vi "WSVCAP SHL Host LL SPI Set Configuration Parameters.vi"(0 "I2C_Clock Divider":u32=20, 11 "error in (no error)":errorcluster) -> (15 "error out":errorcluster)   [LabVIEW 2012]
uses:
  Type Defs/WSVCAP SHL Top Level Control Enum.ctl
  Type Defs/WSVCAP SHL Top Level Control Operation Enum.ctl
  Type Defs/WSVCAP SHL State.ctl
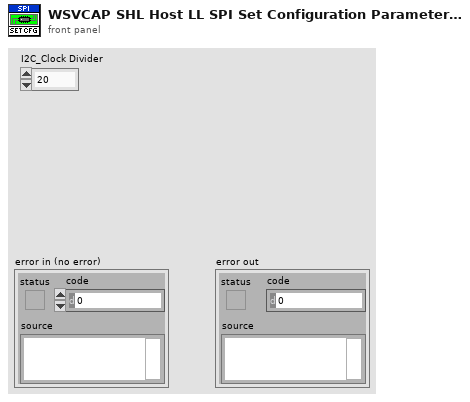
[diagram p1: front panel]
types:
  T1 = typedef "WSVCAP SHL State.ctl" = enum8{"Idle", "Transfer Data"}
  T2 = typedef "WSVCAP SHL Top Level Control Operation Enum.ctl" = enum16{"Initialize", "Set Control", "Read Control", "Close"}
  T3 = typedef "WSVCAP SHL Top Level Control Enum.ctl" = enum16{"Start", "Cmd", "Transaction", "Wait Ticks", "Socket Mask", "UUT Set", "Slave Address", "Sub Address", "Bytes to Write", "Bytes to Read", "Write Data", "Write Flag", "Read Data", "Read Flag", "Ack Read", "Read Status Flag", "Ack Read Status", "Status", "Cycle Count", "Stop Cycle", "Exit"}
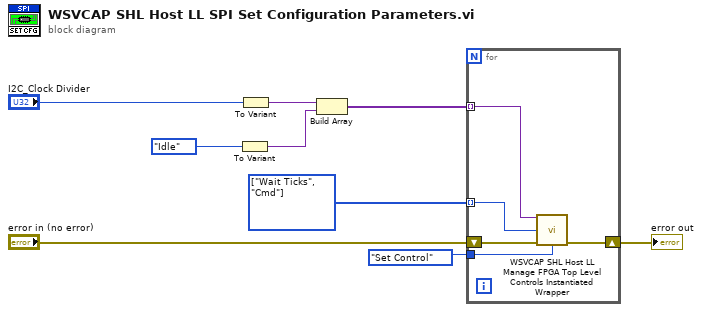
[diagram p0: block diagram]
diagram:
  w4 = T3[] [enum."Wait Ticks", enum."Cmd"] items=["Start", "Cmd", "Transaction", "Wait Ticks", "Socket Mask", "UUT Set", "Slave Address", "Sub Address", "Bytes to Write", "Bytes to Read", "Write Data", "Write Flag", "Read Data", "Read Flag", "Ack Read", "Read Status Flag", "Ack Read Status", "Status", "Cycle Count", "Stop Cycle", "Exit"]
  n1 = To Variant(anything=WSVCAP_SHL_State."Idle" ("SPI_Cmd")) -> (Variant=w1:variant)
  n2 = To Variant(anything="I2C_Clock Divider") -> (Variant=w6:variant)
  n3 = Build Array(w6, w1) -> (w5:variant[])
  n4 = for {
    tunnel: WSVCAP_SHL_Top_Level_Control_Operation_Enum."Set Control" ("Operation") -> [w14]
    tunnel: w5 -> [w13] mode=indexing
    tunnel: w4 -> [w12] mode=indexing
    shift-right: [w10] -> w2
    shift-left: "error in (no error)" -> [w11]
    n5 = call "WSVCAP SHL Host LL Manage FPGA Top Level Controls Instantiated Wrapper.vi"("Value In"=w13, "FPGA Top Level Control"=w12, "error in (no error)"=w11, "Operation"=w14) -> ("error out"=w10:errorcluster)  [unwired: 10 in, 1 out]
  }
  "error out" <- w2
